vi "Status.vi"(8 "error in (no error)":errorcluster, 11 "IKA EUROSTAR Settings in":T1) -> (0 "error out":errorcluster, 1 "Connection Error":bool, 2 "Running":bool, 3 "IKA EUROSTAR Settings Out":T1, 4 "Power":dbl, 5 "Amplitude":dbl)   [LabVIEW 2021, in "IKA EUROSTAR.lvlib"]
uses:
  IKA EUROSTAR.lvlib
  IKA EUROSTAR Settings.ctl
  <vilib>/regexp/Match Regular Expression.xnode
  support/Support Library.lvlib
panel:
  out "read buffer 2":string
  out "read buffer":string
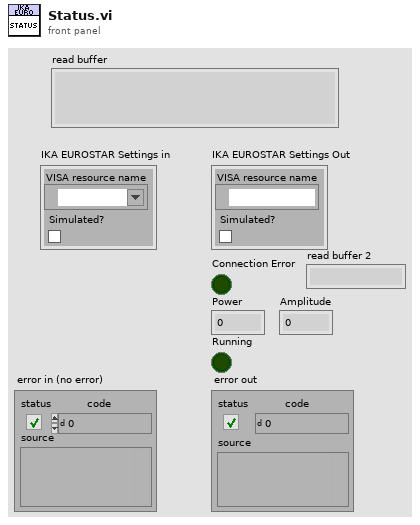
[diagram p1: front panel]
types:
  T1 = typedef "IKA EUROSTAR.lvlib/IKA EUROSTAR Settings.ctl" = cluster{"VISA resource name":refnum<visa-resource-name>, "Simulated?":bool}
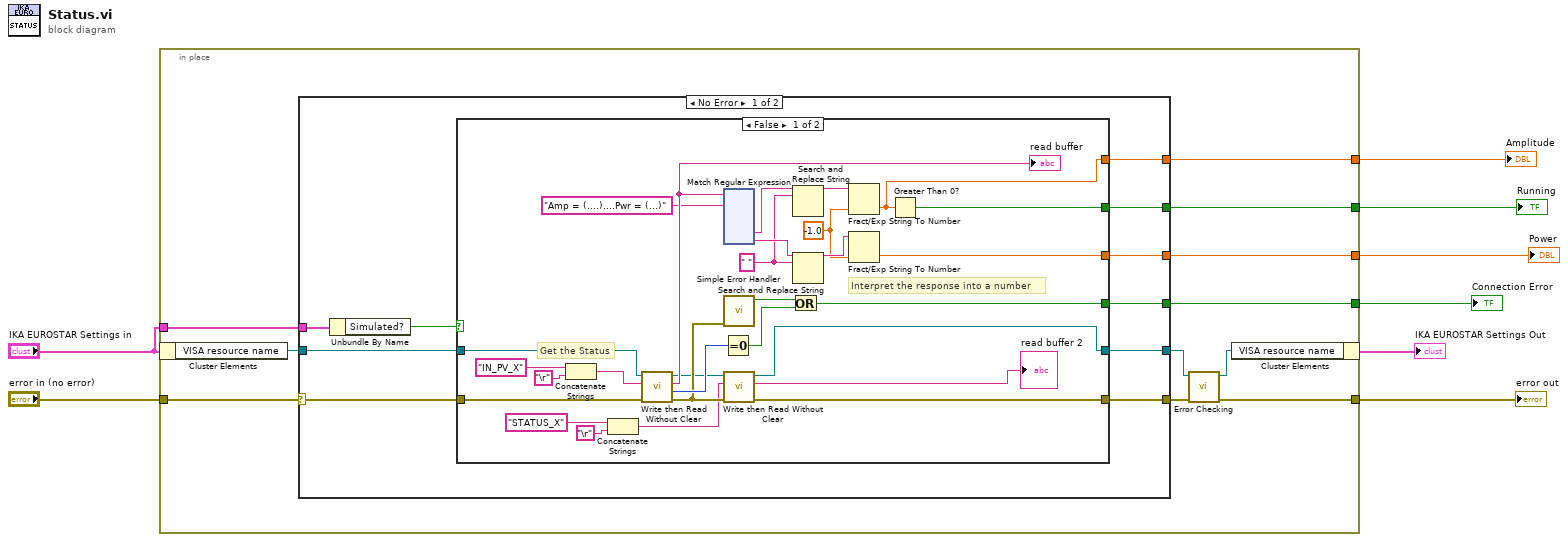
[diagram p0: block diagram]
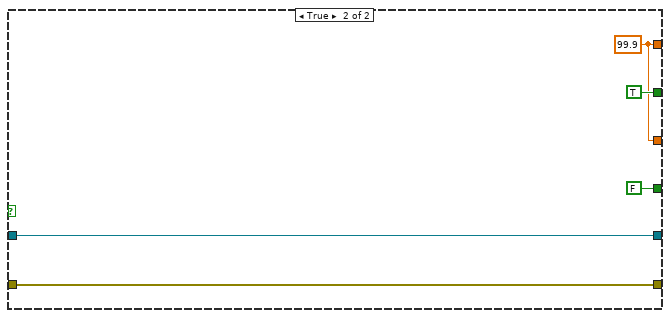
[diagram p2: hidden frame]
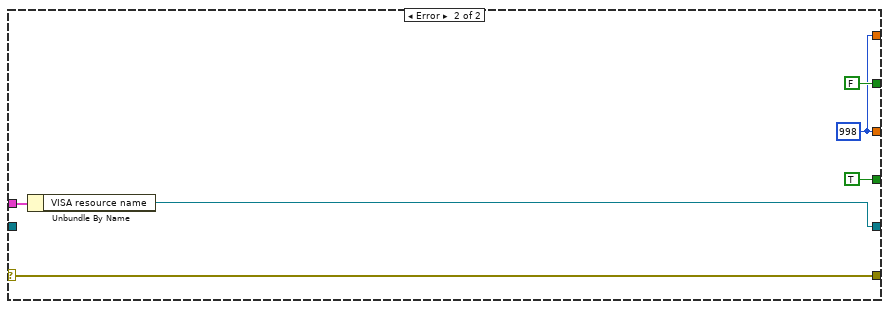
[diagram p3: hidden frame]
diagram:
  n1 = in-place {
    in-place-border: "error in (no error)" -> [w19]
    in-place-border: [w16] -> w7
    in-place-border: "IKA EUROSTAR Settings in" -> [w15]
    in-place-border: [w12] -> w4
    in-place-border: [w10] -> w2
    in-place-border: [w11] -> w3
    in-place-border: [w9] -> w1
    n2 = in-place-cluster #1("IKA EUROSTAR Settings in") -> ("VISA resource name"=w14:refnum<visa-resource-name>)
    n3 = case shown="No Error" w19 {
      selector: w19 -> [w29 w188]
      tunnel: w15 -> [w27 w187]
      tunnel: [w28 w188] -> w17
      tunnel: [w26 w186] -> w18
      tunnel: [w24 TRUE] -> w12
      tunnel: [w23 FALSE] -> w11
      tunnel: w14 -> [w22 _]
      tunnel: [w21 w183] -> w10
      tunnel: [w20 w183] -> w9
      frame No Error {
        n4 = Unbundle By Name(w27) -> ("Simulated?"=w25:bool)
        n5 = case shown="False" w25 {
          tunnel: w29 -> [w55 w182]
          tunnel: [w36 w182] -> w28
          tunnel: [w34 w181] -> w26
          tunnel: w22 -> [w56 w181]
          tunnel: [w52 FALSE] -> w24
          tunnel: [w47 TRUE] -> w23
          tunnel: [w45 w178] -> w21
          tunnel: [w46 w178] -> w20
          frame False {
            w39 = -1.0 ("default (0 DBL)")
            w42 = " " ("search string")
            # "Interpret the response into a number"
            # "Get the Status"
            n6 = Concatenate Strings("IN_PV_X" ("string"), "\r") -> (w48:string)
            n7 = Concatenate Strings("STATUS_X" ("string"), "\r") -> (w30:string)
            n8 = call "Write then Read Without Clear.vi"("error in"=w55, "write buffer"=w48, "VISA resource name in"=w56) -> ("error out"=w37:errorcluster, "Bytes at Port"=w51:u32, "read buffer"=w57:string, "VISA resource name out"=w35:refnum<visa-resource-name>)  [unwired: 5 in]
            "read buffer" <- w57
            n9 = Equal To 0?(x=w51) -> (x = 0?=w50:bool)
            n10 = xnode "Match Regular Expression"("input string"=w57, "regular expression"="Amp = (....)....Pwr = (...)") -> ("submatch 1"=w43:string, "submatch 2"=w44:string)  [unwired: 4 in, 5 out]
            n11 = call <vilib>:"Simple Error Handler.vi"("error in (no error)"=w37) -> ("error?"=w53:bool)  [unwired: 4 in, 4 out]
            n12 = call "Write then Read Without Clear.vi"("error in"=w37, "write buffer"=w30, "VISA resource name in"=w35) -> ("error out"=w36:errorcluster, "read buffer"=→"read buffer 2":string, "VISA resource name out"=w34:refnum<visa-resource-name>)  [unwired: 5 in, 1 out]
            n13 = Or(x=w53, y=w50) -> (x .or. y?=w52:bool)
            n14 = Search and Replace String(input string=w43, search string=w42) -> (result string=w41:string)  [unwired: 6 in, 3 out]
            n15 = Search and Replace String(input string=w44, search string=w42) -> (result string=w40:string)  [unwired: 6 in, 3 out]
            n16 = Fract/Exp String To Number(string=w41, default (0 dbl)=w39) -> (number=w45:dbl)  [unwired: 2 in, 1 out]
            n17 = Fract/Exp String To Number(string=w40, default (0 dbl)=w39) -> (number=w46:dbl)  [unwired: 2 in, 1 out]
            n18 = Greater Than 0?(x=w45) -> (x > 0?=w47:bool)
          }
          frame True {
            w178 = 99.9
          }
        }
      }
      frame Error {
        w183 = 998
        n19 = Unbundle By Name(w187) -> ("VISA resource name"=w186:refnum<visa-resource-name>)
      }
    }
    n20 = call "Error Checking.vi"("error in (no error)"=w17, "VISA resource name"=w18) -> ("error out"=w16:errorcluster, "VISA resource name"=w13:refnum<visa-resource-name>)  [unwired: 7 in, 1 out]
    n21 = in-place-cluster #1("VISA resource name"=w13) -> (→"IKA EUROSTAR Settings Out":T1)
  }
  "error out" <- w7
  "Connection Error" <- w4
  "Power" <- w1
  "Running" <- w3
  "Amplitude" <- w2
